vi "ImportSession.vi"(8 "error in (no error)":errorcluster, 11 "Experiment in":refnum<class "Experiment.lvclass">) -> (0 "error out":errorcluster, 3 "Experiment out":refnum<class "Experiment.lvclass">)   [LabVIEW 2016, in "Experiment.lvclass"]
uses:
  Experiment.lvclass
  Experiment.lvclass/Experiment.ctl
  Database/Database.lvclass
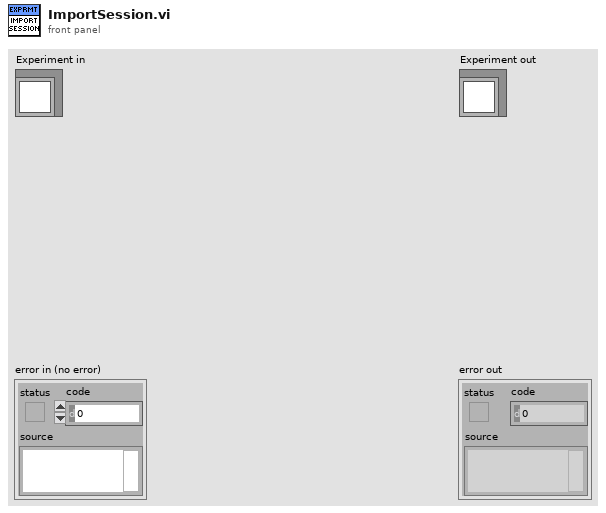
[diagram p1: front panel]
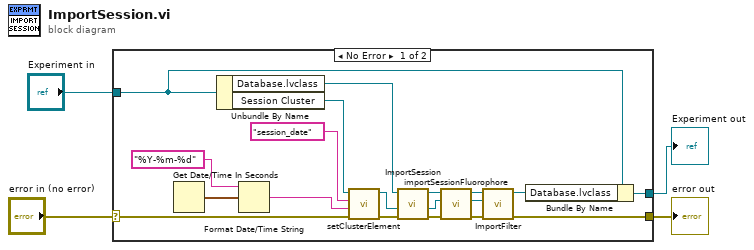
[diagram p0: block diagram]
diagram:
  n1 = case shown="No Error" "error in (no error)" {
    selector: "error in (no error)" -> [w9 w25]
    tunnel: [w15 w25] -> w3
    tunnel: [w22 w24] -> w1
    tunnel: "Experiment in" -> [w5 w24]
    frame No Error {
      n2 = Get Date/Time In Seconds() -> (seconds since 1Jan1904=w13:timestamp)
      n3 = Unbundle By Name(w5) -> ("Database.lvclass"=w23:refnum<class "Database.lvclass">, "Session Cluster"=w11:refnum<vi>)
      n4 = Format Date/Time String(time format string (%c)="%Y-%m-%d", seconds (now)=w13) -> (date/time string=w7:string)  [unwired: 1 out]
      n5 = call "setClusterElement.vi"("error in (no error)"=w9, "Value"=w7, "Label.Text"="session_date", "reference"=w11) -> ("error out"=w8:errorcluster, "reference 2"=w10:refnum<vi>)  [unwired: 6 in]
      n6 = call-dynamic "ImportSession.vi"("error in (no error)"=w8, "Clust Refnum"=w10, "Database in"=w23) -> ("error out"=w19:errorcluster, "Clust Refnum 2"=w20:refnum<vi>, "Database out"=w21:refnum<class "Database.lvclass">)  [unwired: 6 in]
      n7 = call-dynamic "importSessionFluorophore.vi"("error in (no error)"=w19, "Clust Refnum"=w20, "Database in"=w21) -> ("error out"=w16:errorcluster, "Clust Refnum 2"=w17:refnum<vi>, "Database out"=w18:refnum<class "Database.lvclass">)  [unwired: 6 in]
      n8 = call-dynamic "ImportFilter.vi"("error in (no error)"=w16, "Clust Refnum"=w17, "Database in"=w18) -> ("error out"=w15:errorcluster, "Database out"=w14:refnum<class "Database.lvclass">)  [unwired: 6 in, 1 out]
      n9 = Bundle By Name(cluster=w5, "Database.lvclass"=w14) -> (w22:refnum<class "Experiment.lvclass">)
    }
    frame Error {
    }
  }
  "error out" <- w3
  "Experiment out" <- w1
